vi "formula (SubVI).vi"(11 "Table 2":string[][](table)=[["", "50000", "100000", "200000"], ["100", "0", "0", "0"], ["75.3", "-11.3", "-21.7", "-46.55"], ["55.3", "-19.9", "-30.2", "-69.65"], ["35.3", "-30", "-47.2", "-109.2"], ["14.7", "-35.5", "-55.6", "-127.5"], ["10", "-38.8", "-61.8", "-138.6"]]) -> (1 "ArrayFreq":dbl[](array[numeric]), 3 "Array 2":cluster{"X Values":dbl[], "Y Values":dbl[]}[](array[cluster]))   [LabVIEW 2017]
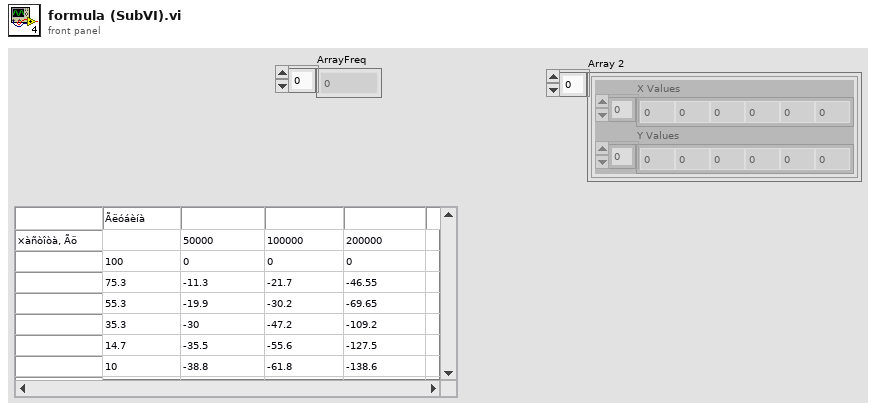
[diagram p1: front panel]
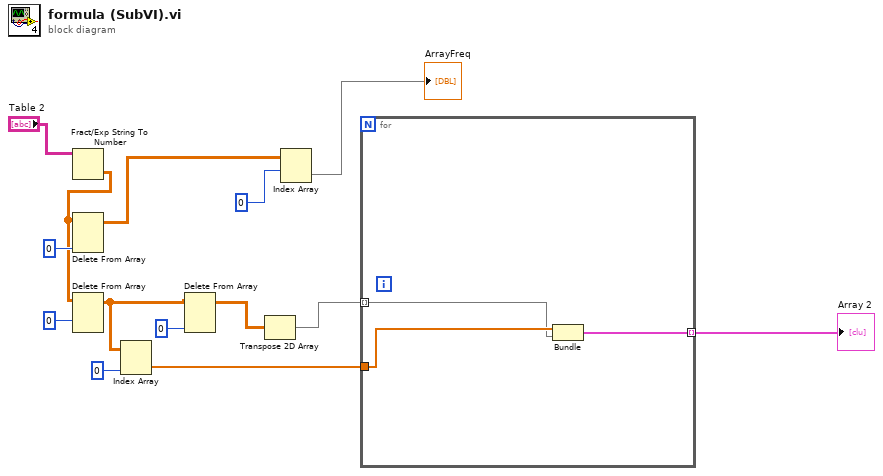
[diagram p0: block diagram]
diagram:
  n1 = Fract/Exp String To Number(string="Table 2") -> (number=w8:dbl[][])  [unwired: 3 in, 1 out]
  n2 = Delete From Array(array=w8, index (col)=0 ("disabled index (col)")) -> (array with subset deleted=w9:dbl[][])  [unwired: 2 in, 1 out]
  n3 = Delete From Array(array=w8, index (row)=0) -> (array with subset deleted=w4:dbl[][])  [unwired: 2 in, 1 out]
  n4 = Index Array(array=w4, index (col)=0 ("disabled index (col)")) -> (element=w3:dbl[])  [unwired: 1 in]
  n5 = Delete From Array(array=w4, index (col)=0) -> (array with subset deleted=w2:dbl[][])  [unwired: 2 in, 1 out]
  n6 = Transpose 2D Array(2D array=w2) -> (transposed array=w1:dbl[][])
  n7 = Index Array(array=w9, index (row)=0) -> (element=→"ArrayFreq":dbl[])  [unwired: 1 in]
  n8 = for {
    tunnel: [w17] -> w14 mode=indexing
    tunnel: w1 -> [w15] mode=indexing
    tunnel: w3 -> [w16]
    n9 = Bundle(w16, w15) -> (w17:cluster{dbl[], dbl[]})  [unwired: 1 in]
  }
  "Array 2" <- w14
